vi "Homing code.vi"() -> ()   [LabVIEW 2020]
panel:
  out "Z position":dbl
  out "Y position":dbl
  in  "stop":bool
  out "Error out":errorcluster={"status"=TRUE, "code"=-2147218439, "source"="Exception occured in SPiiPlusCOM660.AsyncChannel.1: Code 3065, The command cannot be executed while the current motion is in progress in Z Stack Code debug.vi"}
  out "Connected":bool
  out "GetFirmwareVersion 2":string="3.03\r"
  in  "SPIIPLUSCOM660Lib.IAsyncChannel":refnum<k7>
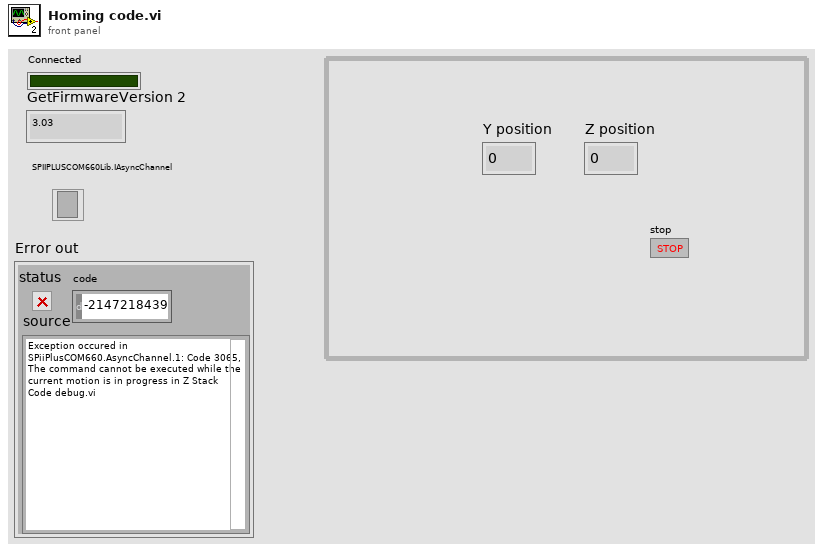
[diagram p1: front panel]
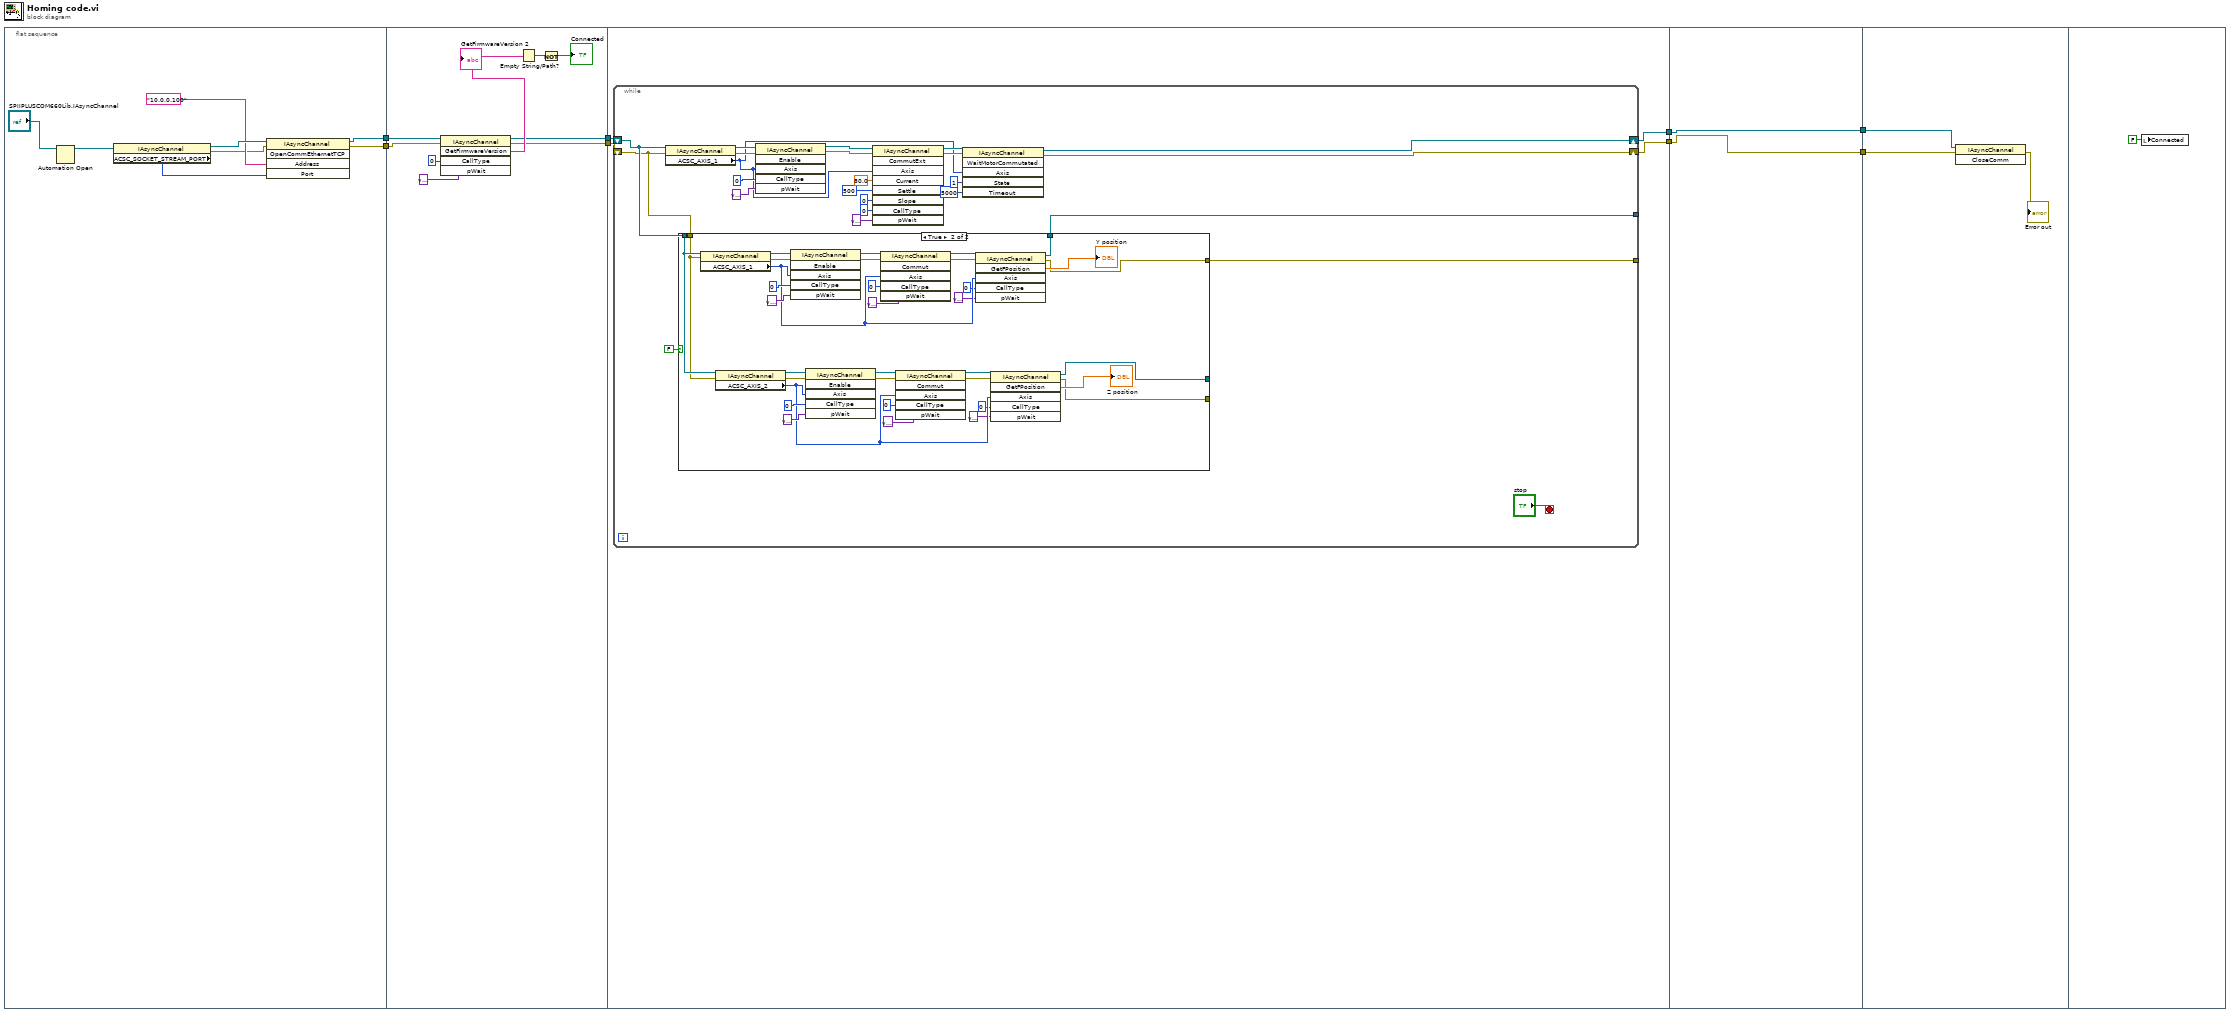
[diagram p0: block diagram]
diagram:
  n1 = flat-sequence {
    tunnel: [w11] -> w8
    tunnel: [w10] -> w7
    tunnel: w8 -> [w21]
    tunnel: w7 -> [w20]
    tunnel: [w18] -> w6
    tunnel: [w17] -> w5
    tunnel: w6 -> [w29]
    tunnel: w5 -> [w28]
    tunnel: [w27] -> w4
    tunnel: [w26] -> w3
    tunnel: w4 -> [w91]
    tunnel: w3 -> [w90]
    tunnel: [w91] -> w2
    tunnel: [w90] -> w1
    tunnel: w2 -> [w93]
    tunnel: w1 -> [w92]
    frame #0 {
      n2 = Automation Open(Automation Refnum="SPIIPLUSCOM660Lib.IAsyncChannel") -> (Automation Refnum=w16:refnum<k7>)  [unwired: 3 in, 1 out]
      n3 = property class="IAsyncChannel"(reference=w16) -> (reference out=w15:refnum<k7>, error out=w9:errorcluster, "ACSC_SOCKET_STREAM_PORT"=w13:i32)  [unwired: 1 in]
      n4 = invoke class="IAsyncChannel" method="OpenCommEthernetTCP"(reference=w15, error in=w9, "Address"="10.0.0.100", "Port"=w13) -> (reference out=w11:refnum<k7>, error out=w10:errorcluster)  [unwired: 1 in, 3 out]
    }
    frame #1 {
      n5 = invoke class="IAsyncChannel" method="GetFirmwareVersion"(reference=w21, error in=w20, "CallType"=u64 0, "pWait"=variant) -> (reference out=w18:refnum<k7>, error out=w17:errorcluster, "GetFirmwareVersion"=w23:string)  [unwired: 1 in, 2 out]
      "GetFirmwareVersion 2" <- w23
      n6 = Empty String/Path?(string/path=w23) -> (empty?=w22:bool)
      n7 = Not(x=w22) -> (.not. x?=→"Connected":bool)
    }
    frame #2 {
      n8 = while {
        shift-right: [w39] -> w27
        shift-left: w29 -> [w46]
        shift-right: [w38] -> w26
        shift-left: w28 -> [w45]
        tunnel: [w42] -> _
        tunnel: [w41] -> _
        stop <- "stop" stop-if-true
        n9 = property class="IAsyncChannel"(reference=w46, error in=w45) -> (reference out=w44:refnum<k7>, error out=w43:errorcluster, "ACSC_AXIS_1"=w37:i32)
        n10 = case shown="True" FALSE {
          tunnel: w46 -> [w54 w65]
          tunnel: w45 -> [w55 w64]
          tunnel: [w54 w59] -> w42
          tunnel: [w55 w58] -> w41
          tunnel: [_ w57] -> _
          tunnel: [_ w56] -> _
          frame False {
          }
          frame True {
            n11 = property class="IAsyncChannel"(reference=w65, error in=w64) -> (reference out=w63:refnum<k7>, error out=w62:errorcluster, "ACSC_AXIS_1"=w81:i32)
            n12 = property class="IAsyncChannel"(reference=w65, error in=w64) -> (reference out=w61:refnum<k7>, error out=w60:errorcluster, "ACSC_AXIS_2"=w69:i32)
            n13 = invoke class="IAsyncChannel" method="Enable"(reference=w63, error in=w62, "Axis"=w81, "CallType"=u64 0, "pWait"=variant) -> (reference out=w87:refnum<k7>, error out=w86:errorcluster)  [unwired: 1 in, 4 out]
            n14 = invoke class="IAsyncChannel" method="Enable"(reference=w61, error in=w60, "Axis"=w69, "CallType"=u64 0, "pWait"=variant) -> (reference out=w75:refnum<k7>, error out=w74:errorcluster)  [unwired: 1 in, 4 out]
            n15 = invoke class="IAsyncChannel" method="Commut"(reference=w87, error in=w86, "Axis"=w81, "CallType"=u64 0, "pWait"=variant) -> (reference out=w83:refnum<k7>, error out=w82:errorcluster)  [unwired: 1 in, 4 out]
            n16 = invoke class="IAsyncChannel" method="Commut"(reference=w75, error in=w74, "Axis"=w69, "CallType"=u64 0, "pWait"=variant) -> (reference out=w71:refnum<k7>, error out=w70:errorcluster)  [unwired: 1 in, 4 out]
            n17 = invoke class="IAsyncChannel" method="GetFPosition"(reference=w83, error in=w82, "Axis"=w81, "CallType"=u64 0, "pWait"=variant) -> (reference out=w59:refnum<k7>, error out=w58:errorcluster, "GetFPosition"=→"Y position":dbl)  [unwired: 1 in, 3 out]
            n18 = invoke class="IAsyncChannel" method="GetFPosition"(reference=w71, error in=w70, "Axis"=w69, "CallType"=u64 0, "pWait"=variant) -> (reference out=w56:refnum<k7>, error out=w57:errorcluster, "GetFPosition"=→"Z position":dbl)  [unwired: 1 in, 3 out]
          }
        }
        n19 = invoke class="IAsyncChannel" method="Enable"(reference=w44, error in=w43, "Axis"=w37, "CallType"=u64 0, "pWait"=variant) -> (reference out=w50:refnum<k7>, error out=w49:errorcluster)  [unwired: 1 in, 4 out]
        n20 = invoke class="IAsyncChannel" method="CommutExt"(reference=w50, error in=w49, "Axis"=w37, "Current"=sgl 80.0, "Settle"=500, "Slope"=0, "CallType"=u64 0, "pWait"=variant) -> (reference out=w48:refnum<k7>, error out=w47:errorcluster)  [unwired: 1 in, 7 out]
        n21 = invoke class="IAsyncChannel" method="WaitMotorCommutated"(reference=w48, error in=w47, "Axis"=w37, "State"=1, "Timeout"=5000) -> (reference out=w39:refnum<k7>, error out=w38:errorcluster)  [unwired: 1 in, 4 out]
      }
    }
    frame #3 {
    }
    frame #4 {
      n22 = invoke class="IAsyncChannel" method="CloseComm"(reference=w93, error in=w92) -> (error out=→"Error out":errorcluster)  [unwired: 1 in, 2 out]
    }
    frame #5 {
      n23 = local write "Connected"(FALSE ("Connected")) -> ()
    }
  }
